vi "Get SMO Serial Number.vi"(8 "error in (no error)":errorcluster, 11 "Instrument.Lockin in":refnum<class "Instrument.Lockin.lvclass">) -> (0 "error out":errorcluster, 2 "Serial Number":string, 3 "Instrument.Lockin out":refnum<class "Instrument.Lockin.lvclass">)   [LabVIEW 2019, in "Instrument.Lockin.lvlib" / "Instrument.Lockin.lvclass"]
doc: "Override this VI to return the serial number of your Instrument"
uses:
  Instrument.Lockin.lvclass
  Instrument.Lockin.lvclass/Instrument.Lockin.ctl
  <userlib>/LevyLab/Instrument Framework/Instrument Types/Lockin/Instrument.LockinAPI.lvclass
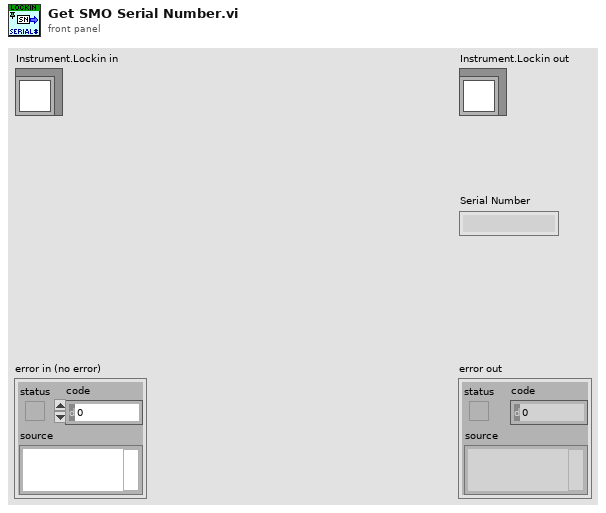
[diagram p1: front panel]
types:
  T1 = typedef "Instrument.Lockin.lvlib/Instrument.DAQ.lvclass/DeviceInfo--Cluster.ctl" = cluster{"DeviceName":string, "DevIsSimulated":bool, "DeviceSerialNumber":u32, "ProductType":string, "ProductCategory":i32, "ProductNumber":u32, "ChassisNumber":u32, "SlotNumber":u32, "ChassisName":string, "ChassisSerialNumber":u32}
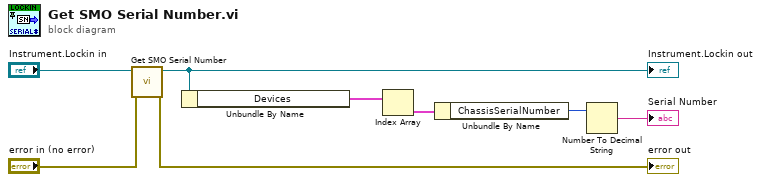
[diagram p0: block diagram]
diagram:
  n1 = call-parent "Get SMO Serial Number.vi"("error in (no error)"="error in (no error)", "Instrument in"="Instrument.Lockin in") -> ("error out"=→"error out":errorcluster, "Instrument out"=w7:refnum<class "Instrument.Lockin.lvclass">)  [unwired: 7 in, 1 out]
  "Instrument.Lockin out" <- w7
  n2 = Unbundle By Name(w7) -> ("Devices"=w3:T1[])
  n3 = Index Array(array=w3) -> (element=w6:T1)  [unwired: 1 in]
  n4 = Unbundle By Name(w6) -> ("ChassisSerialNumber"=w4:u32)
  n5 = Number To Decimal String(number=w4) -> (decimal integer string=→"Serial Number":string)  [unwired: 1 in]
